vi "Cleanup.vi"(0 "Operation Interface in":refnum<class "Program Interface.lvclass">) -> ()   [LabVIEW 2019, in "Program Interface.lvclass"]
uses:
  Program Interface.lvclass
  Program Interface.lvclass/Program Interface.ctl
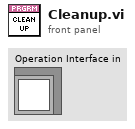
[diagram p1: front panel]
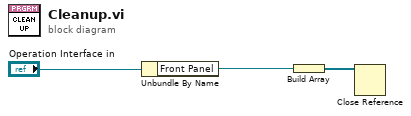
[diagram p0: block diagram]
diagram:
  n1 = Unbundle By Name("Operation Interface in") -> ("Front Panel"=w2:refnum<vi>)
  n2 = Build Array(w2) -> (w1:refnum<vi>[])
  n3 = Close Reference(reference=w1) -> ()  [unwired: 1 in, 1 out]
